vi "NI VeriStand - Set Custom Device Waveform Data Type.vi"(8 "error in (no error)":errorcluster, 10 "Data Type":T1, 11 "Waveform Ref in":T2 format="%.0x") -> (0 "error out":errorcluster, 3 "Waveform Ref out":T2=18446744073709551615 format="%.0x")   [LabVIEW 2026, in "Custom Devices Storage.lvlib"]
uses:
  Custom Devices Storage.lvlib
  <vilib>/NI VeriStand/Custom Device API/Custom Device Item Ref.ctl
  <vilib>/NI VeriStand/Custom Device API/Custom Device Waveform DataType.ctl
  C:/Users/Administrator/Desktop/Jatin/All DNC DLLs/NationalInstruments.VeriStand.SystemDefinitionAPI.dll
  Jatin/All DNC DLLs/NationalInstruments.VeriStand.SystemDefinitionAPI.dll
  <vilib>/NI VeriStand/Custom Device API/Custom Device API.lvlib
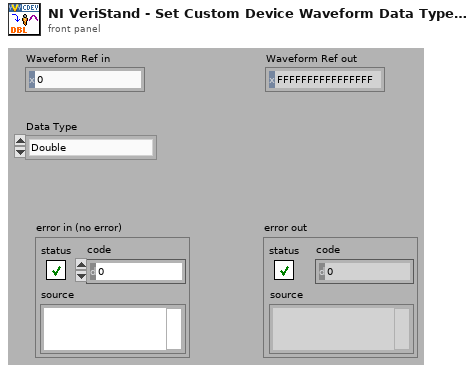
[diagram p1: front panel]
types:
  T1 = typedef "Custom Device API.lvlib/Custom Device Waveform DataType.ctl" = enum16{"Double", "Complex Double"}
  T2 = typedef "Custom Device API.lvlib/Custom Device Item Ref.ctl" = u64
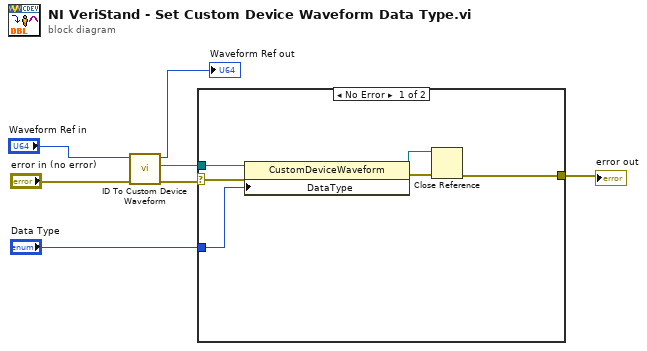
[diagram p0: block diagram]
diagram:
  n1 = call "ID To Custom Device Waveform.vi"("error in (no error)"="error in (no error)", "ID in"="Waveform Ref in") -> ("error out"=w5:errorcluster, "NationalInstruments.VeriStand.SystemDefinitionAPI.CustomDeviceWaveform"=w4:refnum<k39>, "ID out"=→"Waveform Ref out":u64)  [unwired: 7 in]
  n2 = case shown="No Error" w5 {
    selector: w5 -> [w11 w14]
    tunnel: w4 -> [w13 _]
    tunnel: "Data Type" -> [w12 _]
    tunnel: [w8 w14] -> w2
    frame No Error {
      n3 = property class="CustomDeviceWaveform"(reference=w13, error in=w11, "DataType"=w12) -> (reference out=w9:refnum<k39>, error out=w10:errorcluster)
      n4 = Close Reference(reference=w9, error in (no error)=w10) -> (error out=w8:errorcluster)
    }
    frame Error {
    }
  }
  "error out" <- w2
